vi "Read def. var..vi"(11 "settings folder":path) -> (1 "Name column":string[](array[string]), 3 "Default var.":string[][](array[string]))   [LabVIEW 2017]
uses:
  <vilib>/Utility/file.llb/Read Delimited Spreadsheet (string).vi
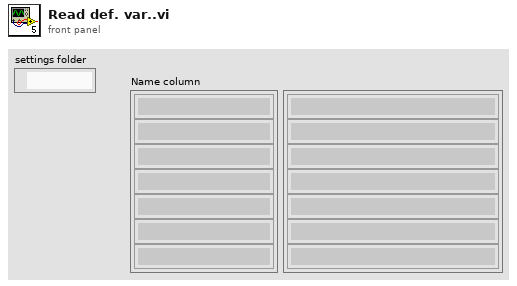
[diagram p1: front panel]
types:
  T1 = enum16{"open", "replace", "create", "open or create", "replace or create", "replace or create with confirmation"}
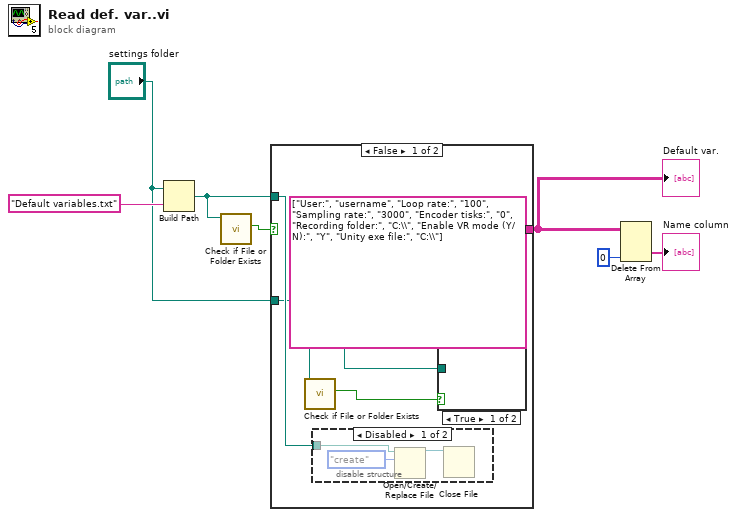
[diagram p0: block diagram]
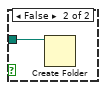
[diagram p2: hidden frame]
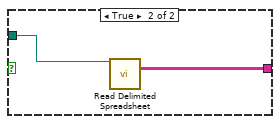
[diagram p4: hidden frame]
diagram:
  n1 = Build Path(base path="settings folder", name or relative path="Default variables.txt") -> (appended path=w3:path)
  n2 = call <vilib>:"Check if File or Folder Exists.vi"("path"=w3) -> ("file or folder exists?"=w2:bool)  [unwired: 8 in, 2 out]
  n3 = case shown="False" w2 {
    tunnel: w3 -> [w10 w17]
    tunnel: [string[][] [["User:", "username"], ["Loop rate:", "100"], ["Sampling rate:", "3000"], ["Encoder tisks:", "0"], ["Recording folder:", "C:\\"], ["Enable VR mode (Y/N):", "Y"], ["Unity exe file:", "C:\\"]] ("Default variables 2") w16] -> w4
    tunnel: "settings folder" -> [w9 _]
    frame False {
      n4 = call <vilib>:"Check if File or Folder Exists.vi"("path"=w9) -> ("file or folder exists?"=w8:bool)  [unwired: 8 in, 2 out]
      n5 = disable-structure shown="Disabled" {
        disable-tunnel: w10 -> [w13 _]
        frame Disabled {
          n6 = Open/Create/Replace File(file path (use dialog)=w13, operation (0:open)=T1."create") -> (refnum out=w14:refnum<file>)  [unwired: 4 in, 2 out]
          n7 = Close File(refnum=w14) -> ()  [unwired: 1 in, 2 out]
        }
        frame Enabled {
        }
      }
      n8 = case shown="True" w8 {
        tunnel: w9 -> [_ w12]
        frame True {
        }
        frame False {
          n9 = Create Folder(path (use dialog)=w12) -> ()  [unwired: 2 in, 3 out]
        }
      }
    }
    frame True {
      n10 = call-poly <vilib>:"Read Delimited Spreadsheet.vi"("file path (dialog if empty)"=w17) -> ("all rows"=w16:string[][])  [unwired: 9 in, 5 out]
    }
  }
  "Default var." <- w4
  n11 = Delete From Array(array=w4, index (col)=0 ("disabled index (col)")) -> (deleted portion=→"Name column":string[])  [unwired: 2 in, 1 out]
